vi "integrate.new.comics.into.collection.vi"() -> ()   [LabVIEW 2024]
uses:
  TypeDefs/comic--cluster.ctl
  <vilib>/addons/_JKI.lib/Serialization/JSON/JKI JSON Serialization.lvlib
  <userlib>/_OpenG.lib/string/string.llb/openg_string.lvlib
panel:
  out "multiples":string[](array[string])
  out "status":string
  out "error out":errorcluster
  in  "comic repo":path=path "D:/Comics/Marvel"
  in  "error in":errorcluster
  in  "path":path=path "D:/Comics/data/comics"
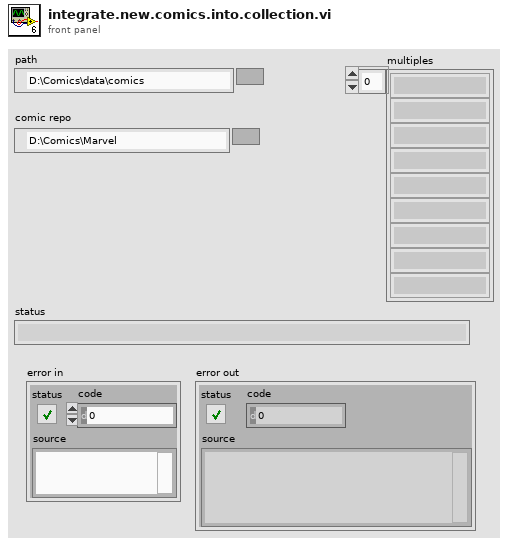
[diagram p1: front panel]
types:
  T1 = typedef "comic--cluster.ctl" = cluster{"id":i32, "digitalId":i32, "title":string, "issueNumber":i32, "variantDescription":string, "description":string, "modified":variant, "upc":string, "format":string, "pageCount":i32, "resourceURI":string, "urls":cluster{"type":string, "url":string}[], "series":cluster{"resourceURI":string, "name":string}, "dates":cluster{"type":string, "date":string}[], "prices":cluster{"price":dbl, "type":string}[], "thumbnail":cluster{"path":string, "extension":string}, "images":cluster{"path":string, "extension":string}[], "creators":cluster{"available":i32, "returned":i32, "collectionURI":string, "items":cluster{"resourceURI":string, "name":string, "role":string}[]}, "characters":cluster{"available":i32, "returned":i32, "collectionURI":string, "items":cluster{"resourceURI":string, "name":string}[]}, "stories":cluster{"available":i32, "returned":i32, "collectionURI":string, "items":cluster{"resourceURI":string, "name":string, "type":string}[]}, "events":cluster{"available":i32, "returned":i32, "collectionURI":string, "items":cluster{"resourceURI":string, "name":string}[]}}
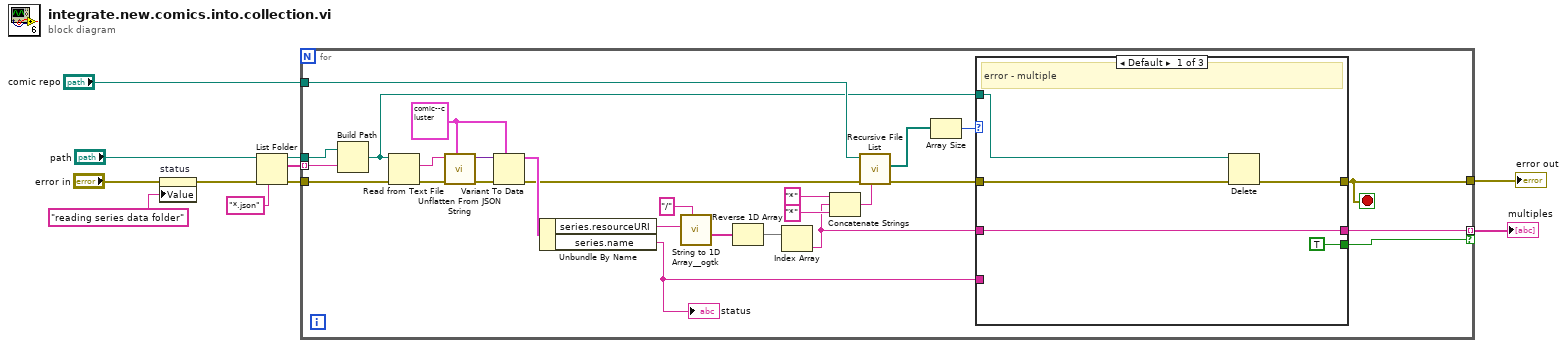
[diagram p0: block diagram]
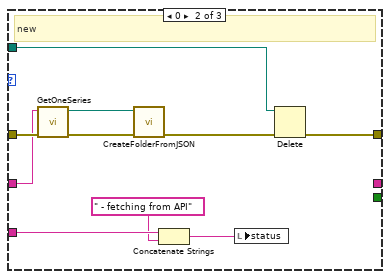
[diagram p2: hidden frame]
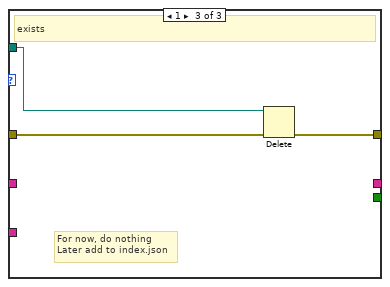
[diagram p3: hidden frame]
diagram:
  n1 = property on="status" class="Str"(error in="error in", "Value"="reading series data folder" ("status")) -> (error out=w2:errorcluster)  [unwired: 1 in, 1 out]
  n2 = List Folder(path="path", pattern="*.json", error in=w2) -> (path out=w7:path, filenames=w8:string[], error out=w9:errorcluster)  [unwired: 1 in, 1 out]
  n3 = for {
    tunnel: w9 -> [w36]
    tunnel: w8 -> [w38] mode=indexing
    tunnel: w7 -> [w37]
    tunnel: "comic repo" -> [w24]
    tunnel: [w17] -> w4
    tunnel: [w15] -> w5 mode=indexing if=w14
    stop <- w17 stop-if-true
    w31 = T1 {"id"=0, "digitalId"=0, "title"="", "issueNumber"=0, "variantDescription"="", "description"="", "modified"=variant, "upc"="", "format"="", "pageCount"=0, "resourceURI"="", "urls"=[], "series"={"resourceURI"="", "name"=""}, "dates"=[], "prices"=[], "thumbnail"={"path"="", "extension"=""}, "images"=[], "creators"={"available"=0, "returned"=0, "collectionURI"="", "items"=[]}, "characters"={"available"=0, "returned"=0, "collectionURI"="", "items"=[]}, "stories"={"available"=0, "returned"=0, "collectionURI"="", "items"=[]}, "events"={"available"=0, "returned"=0, "collectionURI"="", "items"=[]}} ("Cluster")
    n4 = Build Path(base path=w37, name or relative path=w38) -> (appended path=w12:path)
    n5 = Read from Text File(file (use dialog)=w12, error in=w36) -> (text=w34:string, error out=w35:errorcluster)  [unwired: 2 in, 2 out]
    n6 = call <vilib>:"Unflatten From JSON String.vi"("Type and Defaults"=w31, "error in"=w35, "JSON String"=w34) -> ("error out"=w33:errorcluster, "Variant"=w32:variant)  [unwired: 7 in]
    n7 = Variant To Data(error in=w33, type=w31, Variant=w32) -> (data=w30:T1, error out=w25:errorcluster)
    n8 = Unbundle By Name(w30) -> ("series.resourceURI"=w29:string, "series.name"=w13:string)
    "status" <- w13
    n9 = call <userlib>:"String to 1D Array__ogtk.vi"("delimiter (Tab)"="/", "string"=w29) -> ("Array of Strings"=w27:string[])  [unwired: 9 in]
    n10 = Reverse 1D Array(array=w27) -> (reversed array=w26:string[])
    n11 = Index Array(array=w26) -> (element=w16:string)  [unwired: 1 in]
    n12 = Concatenate Strings("*" ("string"), w16, "*" ("string")) -> (w23:string)
    n13 = call <vilib>:"Recursive File List.vi"("pattern"=w23, "error in (no error)"=w25, "Folder Path"=w24) -> ("error out"=w18:errorcluster, "All Files in Dir"=w19:path[])  [unwired: 4 in, 3 out]
    n14 = Array Size(array=w19) -> (size(s)=w20:i32)
    n15 = case shown="Default" w20 {
      tunnel: w18 -> [w41 w53 w56]
      tunnel: [w40 w45 w55] -> w17
      tunnel: w16 -> [w43 w52 _]
      tunnel: [w43 _ _] -> w15
      tunnel: [TRUE _ _] -> w14
      tunnel: w13 -> [_ w49 _]
      tunnel: w12 -> [w39 w44 w54]
      frame Default {
        # "error - multiple"
        n16 = Delete(path (use dialog)=w39, error in=w41) -> (error out=w40:errorcluster)  [unwired: 3 in, 2 out]
      }
      frame 0 {
        # "new"
        n17 = call "GetOneSeries.vi"("error in (no error)"=w53, "id"=w52) -> ("error out"=w50:errorcluster, "last path"=w51:path)  [unwired: 8 in]
        n18 = call "CreateFolderFromJSON.vi"("error in"=w50, "json file path"=w51) -> ("error out"=w46:errorcluster)  [unwired: 9 in]
        n19 = Concatenate Strings(w49, " - fetching from API") -> (w47:string)
        n20 = local write "status"(w47) -> ()
        n21 = Delete(path (use dialog)=w44, error in=w46) -> (error out=w45:errorcluster)  [unwired: 3 in, 2 out]
      }
      frame 1 {
        # "For now, do nothing\nLater add to index.json"
        # "exists"
        n22 = Delete(path (use dialog)=w54, error in=w56) -> (error out=w55:errorcluster)  [unwired: 3 in, 2 out]
      }
    }
  }
  "error out" <- w4
  "multiples" <- w5
